vi "IniDrive4Spark.vi"(3 "refnum name":string="RobotDrive", 5 "Left Motor Inverted":bool, 7 "Right Motor Inverted":bool, 8 "Motor4":T1=enum."Invalid", 9 "Motor3":T1=enum."Invalid", 10 "Motor2":T1=enum."Invalid", 11 "Motor1":T1=enum."Invalid") -> ()   [LabVIEW 2016]
uses:
  <vilib>/Rock Robotics/SystemInterfaces/DIO/FPGA_DIOPWMChannel.ctl
  <vilib>/Rock Robotics/WPI/SafetyOutput/WPI_SafetyOutputConfigMenu.ctl
  <vilib>/Rock Robotics/WPI/RobotDrive/WPI_RobotDriveOpen4MotorWithSPARK.vi
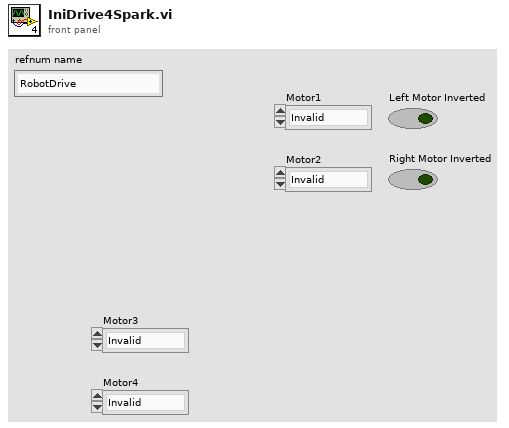
[diagram p1: front panel]
types:
  T1 = typedef "FPGA_DIOPWMChannel.ctl" = enum8{"PWM 0", "PWM 1", "PWM 2", "PWM 3", "PWM 4", "PWM 5", "PWM 6", "PWM 7", "PWM 8", "PWM 9", "PWM MXP 0", "PWM MXP 1", "PWM MXP 2", "PWM MXP 3", "PWM MXP 4", "PWM MXP 5", "PWM MXP 6", "PWM MXP 7", "PWM MXP 8", "PWM MXP 9", "Invalid"}
  T2 = typedef "WPI_SafetyOutputConfigMenu.ctl" = enum16{"Enable", "Disable"}
  T3 = typedef "WPI_RobotDriveDevRef.ctl" = cluster{"DevStatus":errorcluster, "Motors[]":T4[], "Square Inputs":bool, "Max Output":dbl}
  T4 = typedef "WPI_MotorControlDeviceRef.ctl" = cluster{"DeviceStatus":errorcluster, "Type":T5, "PWM":cluster{"PWM Channel":T1, "DeadBand":T6}, "CAN":cluster{"Device Number":u8, "SetOutput VI Ref":variant, "GetOutput VI Ref":variant, "Enable VI Ref":variant, "Disable VI Ref":variant, "Data":variant}, "Invert":bool}
  T5 = typedef "WPI_MotorControlType.ctl" = enum16{"PWM", "CAN"}
  T6 = typedef "WPI_PWMDeadband.ctl" = cluster{"Name":string, "maxPositivePwm":i32, "minPositivePwm":i32, "centerPwm":i32, "maxNegativePwm":i32, "minNegativePwm":i32, "angularRange":u16}
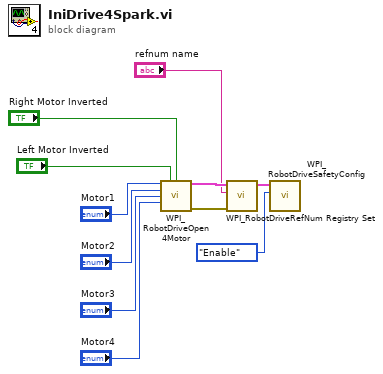
[diagram p0: block diagram]
diagram:
  n1 = call-poly <vilib>:"WPI_RobotDriveOpen4Motor.vi"("Rear Left Motor"="Motor1", "Rear Left Motor Inverted"="Left Motor Inverted", "Rear Right Motor Inverted"="Right Motor Inverted", "Rear Right Motor"="Motor2", "Front Left Motor"="Motor3", "Front Right Motor"="Motor4") -> ("RobotDriveDevRef"=w11:T3, "error out"=w10:errorcluster)  [unwired: 8 in]
  n2 = call <vilib>:"WPI_RobotDriveRefNum Registry Set.vi"("error in (no error)"=w10, "refnum name"="refnum name", "RobotDriveDevRef"=w11) -> ("RobotDriveDevRef"=w9:T3)  [unwired: 1 in, 7 out]
  n3 = call <vilib>:"WPI_RobotDriveSafetyConfig.vi"("mode"=WPI_SafetyOutputConfigMenu."Enable", "RobotDriveDevRef"=w9) -> ()  [unwired: 8 in, 2 out]
